vi "Parameter_1st_part.vi"(0 "S":dbl[](array[numeric]), 1 "测试":bool, 5 "A\\B":dbl[](array[numeric]), 7 "Correction Data 1st":dbl[](array[numeric]), 9 "Biometry Configuration":T1, 11 "Error In":errorcluster caption="错误输入") -> (3 "晶体最值位置":dbl, 4 "角膜厚度":dbl, 6 "开始位置":dbl, 8 "晶体厚度":dbl, 10 "最值位置":dbl, 14 "前方深度":dbl, 15 "Error Out":errorcluster caption="错误输出")   [LabVIEW 2015, in "Boimetry Processing.lvlib"]
doc: "计算眼前节的结果"
uses:
  Boimetry Processing.lvlib
  Controls/Biometry Configuration.ctl
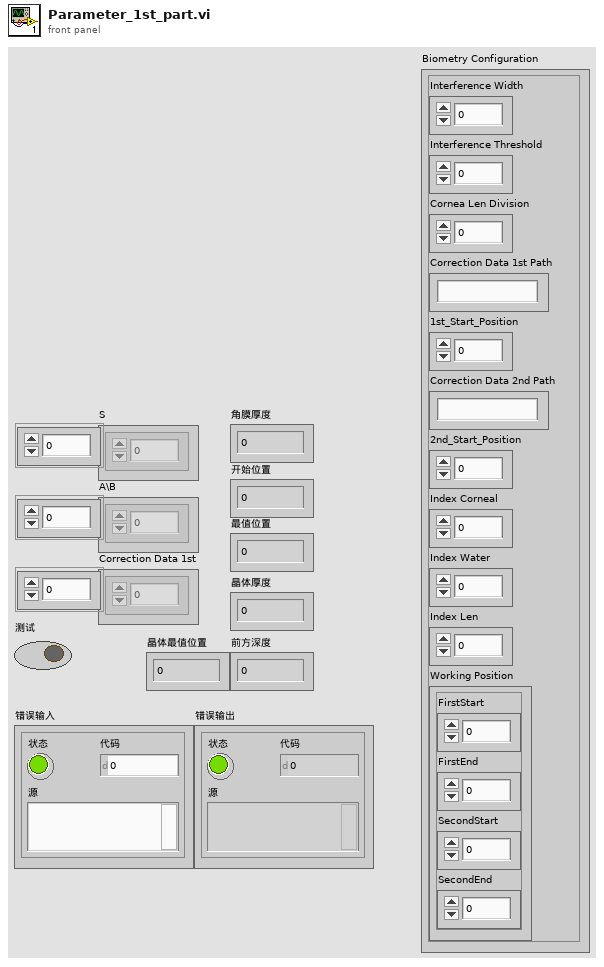
[diagram p1: front panel]
types:
  T1 = typedef "Boimetry Processing.lvlib/Biometry Configuration.ctl" = cluster{"Interference Width":i32, "Interference Threshold":dbl, "Cornea Len Division":i32, "Correction Data 1st Path":string, "1st_Start_Position":dbl, "Correction Data 2nd Path":string, "2nd_Start_Position":dbl, "Index Corneal":dbl, "Index Water":dbl, "Index Len":dbl, "Working Position":cluster{"FirstStart":i32, "FirstEnd":i32, "SecondStart":i32, "SecondEnd":i32}}
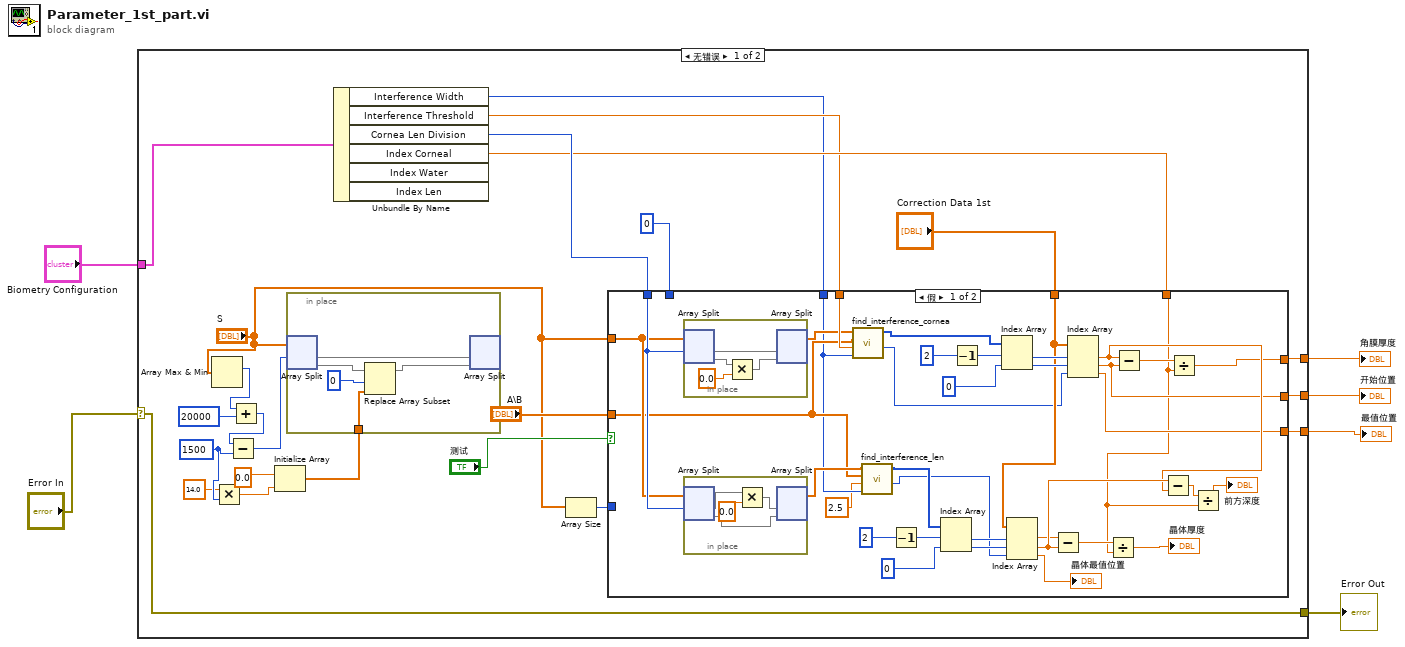
[diagram p0: block diagram]
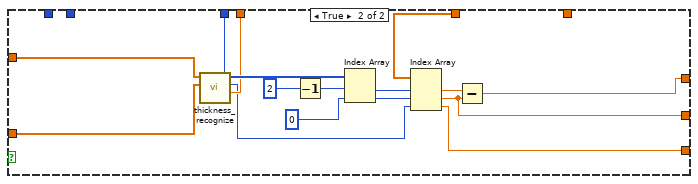
[diagram p2: hidden frame]
diagram:
  n1 = case shown="无错误" "Error In" {
    selector: "Error In" -> [w13 w96]
    tunnel: [w26 _] -> w6
    tunnel: [w25 _] -> w5
    tunnel: [w24 _] -> w4
    tunnel: [w13 w96] -> w2
    tunnel: "Biometry Configuration" -> [w12 _]
    frame No Error {
      w21 = 1500 ("y")
      n2 = Array Max & Min(array="S") -> (max index (indices)=w17:i32)  [unwired: 3 out]
      n3 = Multiply(x=14.0, y=w21) -> (x*y=w22:dbl)
      n4 = Add(x=w17, y=20000) -> (x+y=w18:i32)
      n5 = Subtract(x=w18, y=w21) -> (x-y=w16:i32)
      n6 = Initialize Array(0.0 ("元素"), w22) -> (w15:dbl[])
      n7 = in-place {
        in-place-border: w15 -> [w32]
        n8 = in-place-split #1("S", w16) -> (w35:dbl[], w33:dbl[])
        n9 = Replace Array Subset(array=w33, new element=w32, index=0 ("索引")) -> (w31:dbl[])
        n10 = in-place-split #1(w35, w31) -> ()  [unwired: 2 out]
      }
      n11 = Unbundle By Name(w12) -> ("Interference Width"=w7:i32, "Interference Threshold"=w8:dbl, "Cornea Len Division"=w11:i32, "Index Corneal"=w9:dbl)  [unwired: 2 out]
      n12 = Array Size(array="S") -> (size(s)=w28:i32)
      n13 = case shown="假" "测试" {
        tunnel: "A\\B" -> [w43 w84]
        tunnel: 0 ("索引") -> [_ _]
        tunnel: w11 -> [w50 _]
        tunnel: w28 -> [_ _]
        tunnel: "S" -> [w46 w85]
        tunnel: w9 -> [w37 _]
        tunnel: "Correction Data 1st" -> [w65 w88]
        tunnel: w8 -> [w49 w83]
        tunnel: w7 -> [w42 w82]
        tunnel: [w61 w87] -> w26
        tunnel: [w60 w86] -> w25
        tunnel: [w59 w80] -> w24
        frame False {
          n14 = in-place {
            n15 = in-place-split #2(w46, w50) -> (w79:dbl[], w77:dbl[])
            n16 = Multiply(x=w77, y=0.0) -> (x*y=w76:dbl[])
            n17 = in-place-split #2(w79, w76) -> (w45:dbl[])  [unwired: 1 out]
          }
          n18 = in-place {
            n19 = in-place-split #3(w46, w50) -> (w74:dbl[], w72:dbl[])
            n20 = Multiply(x=w74, y=0.0) -> (x*y=w73:dbl[])
            n21 = in-place-split #3(w73, w72) -> (w44:dbl[])  [unwired: 1 out]
          }
          n22 = call "find_interference_cornea.vi"("干涉长度"=w42, "阈值"=w49, "A"=w43, "S"=w45) -> ("Max_Index"=w47:i32, "INDEX"=w48:i32[])  [unwired: 5 in, 1 out]
          n23 = call "find_interference_len.vi"("干涉长度"=w42, "阈值"=2.5, "A"=w43, "S"=w44) -> ("Max_Index"=w39:i32, "INDEX"=w40:i32[])  [unwired: 5 in, 1 out]
          n24 = Decrement(x=2) -> (x-1=w55:i32)
          n25 = Index Array(array=w40, index #1=w55, index #2=0 ("索引")) -> (element #1=w57:i32, element #2=w56:i32)
          n26 = Decrement(x=2) -> (x-1=w68:i32)
          n27 = Index Array(array=w48, index #1=w68, index #2=0 ("索引")) -> (element #1=w70:i32, element #2=w69:i32)
          n28 = Index Array(array=w65, index #1=w57, index #2=w56, index #3=w39) -> (element #1=w53:dbl, element #2=w63:dbl, element #3=→"晶体最值位置":dbl)
          n29 = Subtract(x=w53, y=w63) -> (x-y=w52:dbl)
          n30 = Index Array(array=w65, index #1=w70, index #2=w69, index #3=w47) -> (element #1=w62:dbl, element #2=w60:dbl, element #3=w59:dbl)
          n31 = Divide(x=w52, y=w37) -> (x/y=→"晶体厚度":dbl)
          n32 = Subtract(x=w62, y=w60) -> (x-y=w66:dbl)
          n33 = Subtract(x=w63, y=w62) -> (x-y=w38:dbl)
          n34 = Divide(x=w66, y=w37) -> (x/y=w61:dbl)
          n35 = Divide(x=w38, y=w37) -> (x/y=→"前方深度":dbl)
        }
        frame True {
          n36 = call "thickness_recognize.vi"("干涉宽度"=w82, "干涉阈值"=w83, "A"=w84, "S"=w85) -> ("MAX_Index"=w81:i32, "INDEX"=w90:i32[])  [unwired: 5 in, 1 out]
          n37 = Decrement(x=2) -> (x-1=w92:i32)
          n38 = Index Array(array=w90, index #1=w92, index #2=0 ("索引")) -> (element #1=w94:i32, element #2=w93:i32)
          n39 = Index Array(array=w88, index #1=w94, index #2=w93, index #3=w81) -> (element #1=w89:dbl, element #2=w86:dbl, element #3=w80:dbl)
          n40 = Subtract(x=w89, y=w86) -> (x-y=w87:dbl)
        }
      }
    }
    frame Error {
    }
  }
  "角膜厚度" <- w6
  "开始位置" <- w5
  "最值位置" <- w4
  "Error Out" <- w2
